vi "getLockStatus.vi"(8 "error in":errorcluster, 11 "connection ID":i32) -> (0 "error out":errorcluster, 1 "authorized":bool, 2 "locked":bool, 3 "connection ID":i32)   [LabVIEW 2016]
doc: "This function returns if the device is locked and if the current client is authorized to use the device."
panel:
  out "params_cluster":cluster{"Numeric":i32}
  in  "Params_cluster":cluster{"Numeric":dbl}
  in  "results_cluster":T1
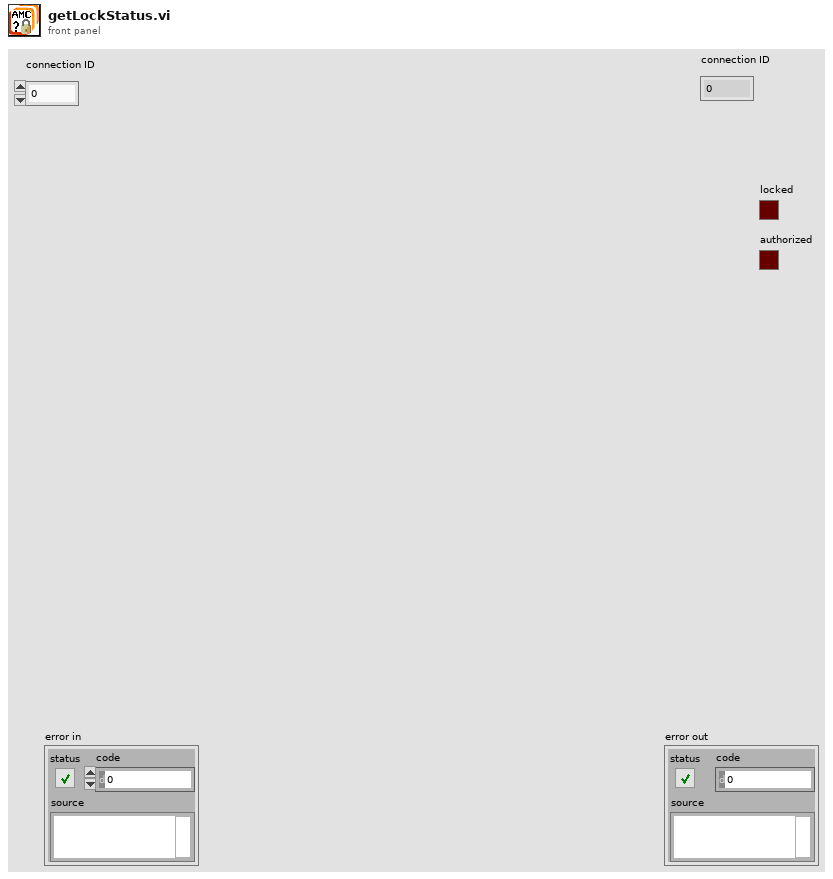
[diagram p1: front panel]
types:
  T1 = cluster{"errNo":i32, "locked":bool, "authorized":bool}
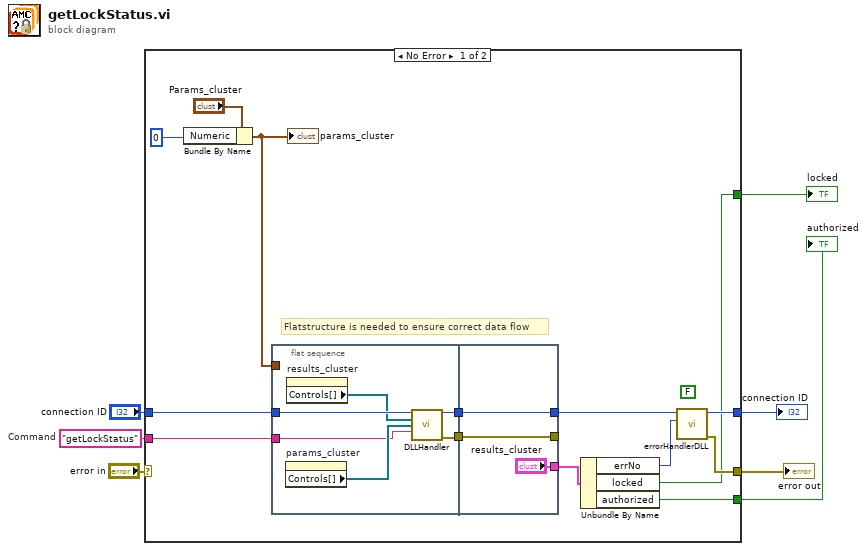
[diagram p0: block diagram]
diagram:
  w5 = "getLockStatus"  # Command
  n1 = case shown="No Error" "error in" {
    selector: "error in" -> [_ w32]
    tunnel: [w11 w32] -> w7
    tunnel: "connection ID" -> [w21 w31]
    tunnel: w5 -> [w18 _]
    tunnel: [w13 w31] -> w3
    tunnel: [w9 _] -> w2
    tunnel: [w8 _] -> w1
    frame No Error {
      (unwired) FALSE ("show popup")
      # "Flatstructure is needed to ensure correct data flow"
      n2 = Bundle By Name(cluster="Params_cluster", "Numeric"=0) -> (w16:cluster{"Numeric":dbl})
      "params_cluster" <- w16
      n3 = flat-sequence {
        tunnel: w21 -> [w27]
        tunnel: w18 -> [w24]
        tunnel: [w23] -> w17
        tunnel: w16 -> [_]
        tunnel: [w22] -> w14
        tunnel: ["results_cluster"] -> w20
        tunnel: [w30] -> w15
        tunnel: [w28] -> _
        tunnel: w17 -> [w28]
        tunnel: w14 -> [w30]
        frame #0 {
          n4 = property on="params_cluster" class="Clust (strict)"() -> ("Controls[]"=w25:refnum<vi>[])  [unwired: 2 in, 2 out]
          n5 = property on="results_cluster" class="Clust (strict)"() -> ("Controls[]"=w26:refnum<vi>[])  [unwired: 2 in, 2 out]
          n6 = call "DLLHandler.vi"("connection ID"=w27, "results_cluster"=w26, "params_cluster"=w25, "method"=w24) -> ("connection ID out"=w22:i32, "error"=w23:errorcluster)  [unwired: 10 in]
        }
        frame #1 {
        }
      }
      n7 = Unbundle By Name(w20) -> ("errNo"=w12:i32, "locked"=w9:bool, "authorized"=w8:bool)
      n8 = call "errorHandlerDLL.vi"("error number"=w12, "connection ID"=w15) -> ("error out"=w11:errorcluster, "connection ID"=w13:i32)  [unwired: 8 in]
    }
    frame Error {
    }
  }
  "error out" <- w7
  "connection ID" <- w3
  "locked" <- w2
  "authorized" <- w1
